vi "proc_wait.vi"(4 "error in":errorcluster, 6 "vars runtime":T2, 7 "vars general":T1) -> (0 "error out":errorcluster, 2 "vars runtime":T2, 3 "vars general":T1)   [LabVIEW 2015]
uses:
  Type Definitions/vars_runtime.ctl
  Type Definitions/vars_settings.ctl
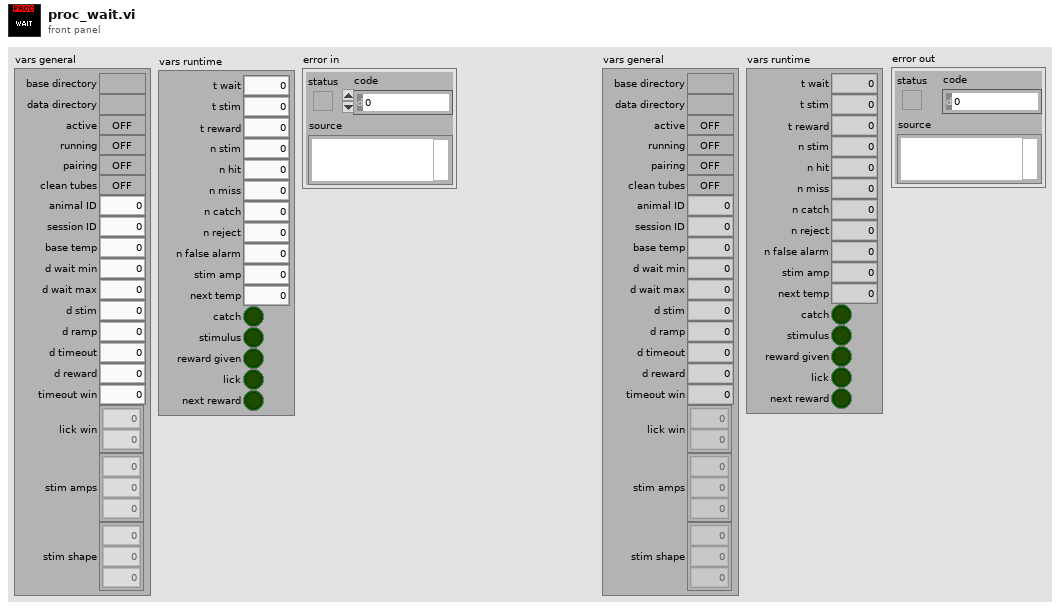
[diagram p1: front panel]
types:
  T1 = typedef "vars_settings.ctl" = cluster{"base directory":path, "data directory":path, "active":bool, "running":bool, "pairing":bool, "clean tubes":bool, "animal ID":u16, "session ID":u16, "base temp":sgl, "d wait min":u16, "d wait max":u16, "d stim":u16, "d ramp":u16, "d timeout":u16, "d reward":u16, "timeout win":u16, "lick win":i32[], "stim amps":dbl[], "stim shape":dbl[]}
  T2 = typedef "vars_runtime.ctl" = cluster{"t wait":u16, "t stim":u16, "t reward":u16, "n stim":u16, "n hit":u16, "n miss":u16, "n catch":u16, "n reject":u16, "n false alarm":u16, "stim amp":sgl, "next temp":sgl, "catch":bool, "stimulus":bool, "reward given":bool, "lick":bool, "next reward":bool}
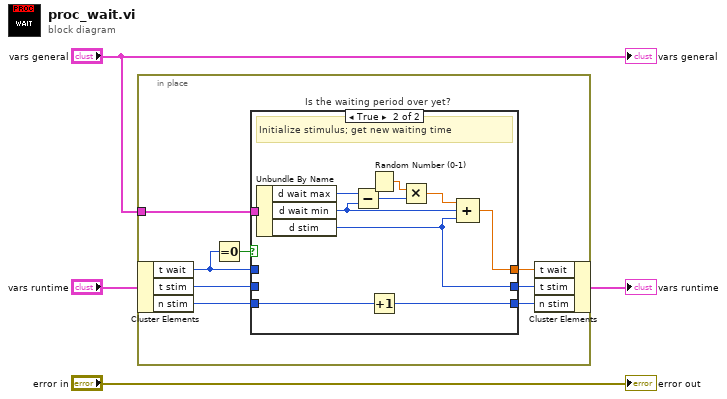
[diagram p0: block diagram]
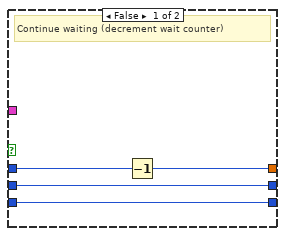
[diagram p2: hidden frame]
diagram:
  n1 = in-place {
    in-place-border: "vars general" -> [w6]
    n2 = in-place-cluster #1("vars runtime") -> ("t wait"=w10:u16, "t stim"=w9:u16, "n stim"=w11:u16)
    n3 = Equal To 0?(x=w10) -> (x = 0?=w12:bool)
    n4 = case "Is the waiting period over yet?" shown="True" w12 {
      tunnel: w10 -> [w16 _]
      tunnel: [w15 w18] -> w8
      tunnel: w9 -> [w14 _]
      tunnel: w11 -> [w13 w26]
      tunnel: [w13 w25] -> w5
      tunnel: [w14 w19] -> w7
      tunnel: w6 -> [_ w21]
      frame False {
        # "Continue waiting (decrement wait counter)"
        n5 = Decrement(x=w16) -> (x-1=w15:u16)
      }
      frame True {
        # "Initialize stimulus; get new waiting time"
        n6 = Unbundle By Name(w21) -> ("d wait max"=w20:u16, "d wait min"=w17:u16, "d stim"=w19:u16)
        n7 = Subtract(x=w20, y=w17) -> (x-y=w24:u16)
        n8 = Random Number (0-1)() -> (number: 0 to 1=w23:dbl)
        n9 = Increment(x=w26) -> (x+1=w25:u16)
        n10 = Multiply(x=w23, y=w24) -> (x*y=w22:dbl)
        n11 = Compound Arithmetic op=ADD(w22, w17, w19) -> (w18:dbl)
      }
    }
    n12 = in-place-cluster #1("t wait"=w8, "t stim"=w7, "n stim"=w5) -> (→"vars runtime":T2)
  }
  "vars general" <- "vars general"
  "error out" <- "error in"
